vi "GetData.vi"(8 "error in (no error)":errorcluster, 11 "BME68x in":refnum<class "BME680.lvclass">) -> (0 "error out":errorcluster, 3 "BME68x out":refnum<class "BME680.lvclass">)   [LabVIEW 2022 SP3, in "BME680.lvlib" / "BME680.lvclass"]
uses:
  BME680.lvclass
  BME680.lvclass/BME680.ctl
panel:
  in  "Opmode":i32
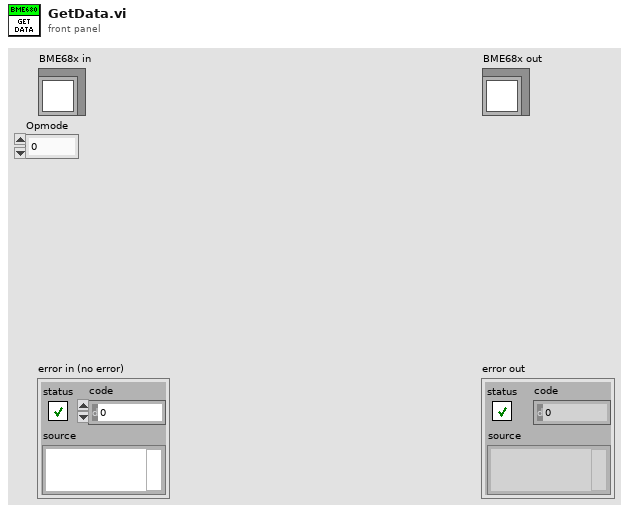
[diagram p1: front panel]
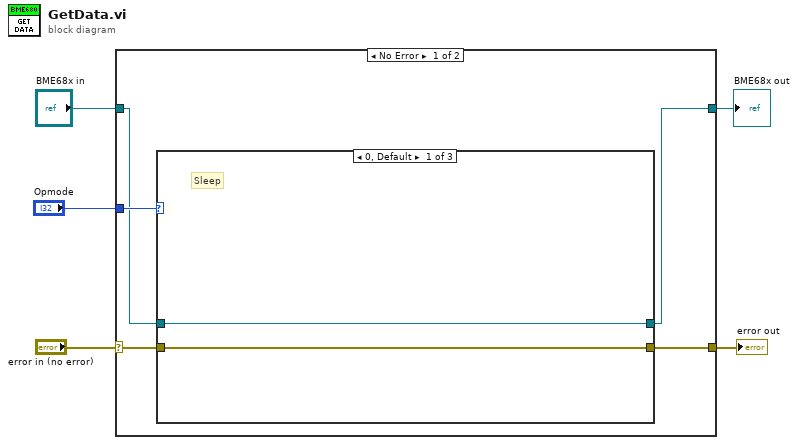
[diagram p0: block diagram]
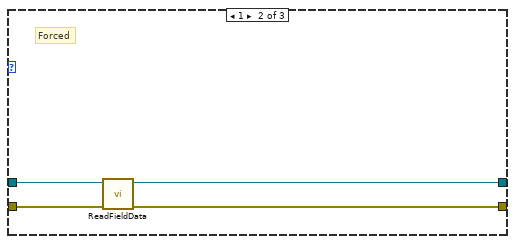
[diagram p2: hidden frame]
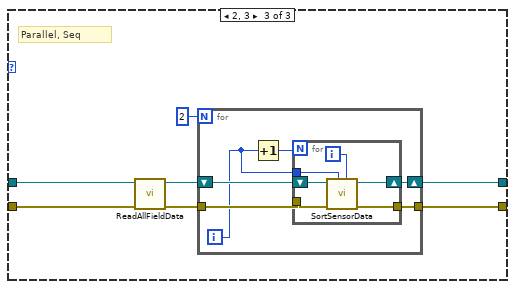
[diagram p3: hidden frame]
diagram:
  n1 = case shown="No Error" "error in (no error)" {
    selector: "error in (no error)" -> [w10 w37]
    tunnel: [w9 w37] -> w4
    tunnel: [w6 w36] -> w2
    tunnel: "BME68x in" -> [w7 w36]
    tunnel: "Opmode" -> [w8 _]
    frame No Error {
      n2 = case shown="0, Default" w8 {
        tunnel: w10 -> [w12 w16 w23]
        tunnel: [w12 w14 w18] -> w9
        tunnel: w7 -> [w11 w15 w22]
        tunnel: [w11 w13 w17] -> w6
        frame 0, Default {
          # "Sleep"
        }
        frame 1 {
          # "Forced"
          n3 = call "ReadFieldData.vi"("error in (no error)"=w16, "BME68x in"=w15) -> ("error out"=w14:errorcluster, "BME68x out"=w13:refnum<class "BME680.lvclass">)  [unwired: 8 in]
        }
        frame 2, 3 {
          # "Parallel, Seq"
          n4 = call "ReadAllFieldData.vi"("error in (no error)"=w23, "BME68x in"=w22) -> ("error out"=w21:errorcluster, "BME68x out"=w20:refnum<class "BME680.lvclass">)  [unwired: 8 in]
          n5 = for {
            N: 2 -> [_]
            tunnel: w21 -> [w29]
            tunnel: [w26] -> w18
            shift-right: [w25] -> w17
            shift-left: w20 -> [w28]
            i -> [w24]
            n6 = Increment(x=w24) -> (x+1=w27:i32)
            n7 = for {
              N: w27 -> [_]
              tunnel: w29 -> [w35]
              tunnel: [w33] -> w26
              tunnel: w24 -> [w31]
              shift-right: [w32] -> w25
              shift-left: w28 -> [w34]
              i -> [w30]
              n8 = call "SortSensorData.vi"("index_high"=w30, "index_low"=w31, "error in (no error)"=w35, "BME68x in"=w34) -> ("error out"=w33:errorcluster, "BME68x out"=w32:refnum<class "BME680.lvclass">)  [unwired: 6 in]
            }
          }
        }
      }
    }
    frame Error {
    }
  }
  "error out" <- w4
  "BME68x out" <- w2
